vi "Division of Complex Polynomials.vi"(2 "Q":cdb[](array[numeric]) format="%.2f", 3 "P":cdb[](array[numeric]) format="%.2f") -> (0 "Rest":cdb[](array[numeric]) format="%.2f", 1 "P/Q":cdb[](array[numeric]) format="%.2f")   [LabVIEW 2020, in "NI_AdvCtrl_continuous linear.lvlib"]
doc: "LabVIEW no longer supports this VI. You can obtain similar functionality by installing the LabVIEW Simulation Module."
uses:
  <vilib>/addons/control/advanced/NI_AdvCtrl_continuous linear.lvlib
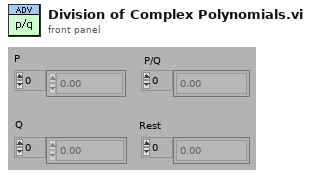
[diagram p1: front panel]
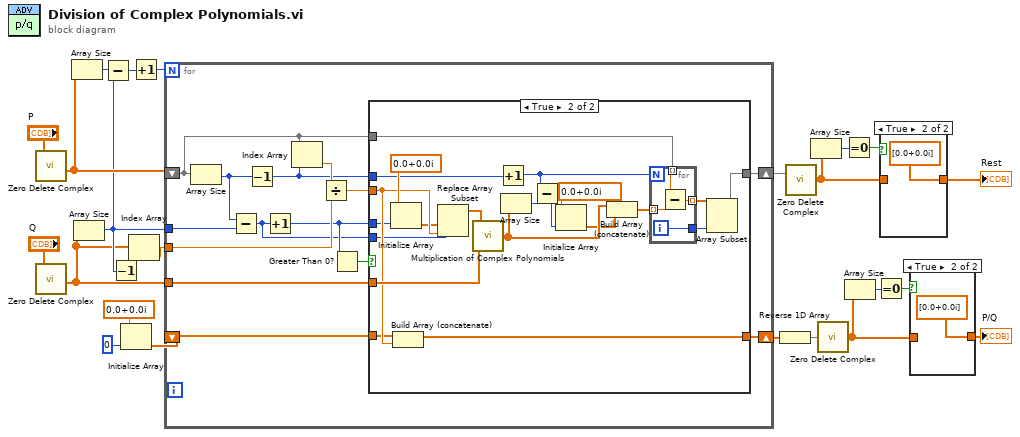
[diagram p0: block diagram]
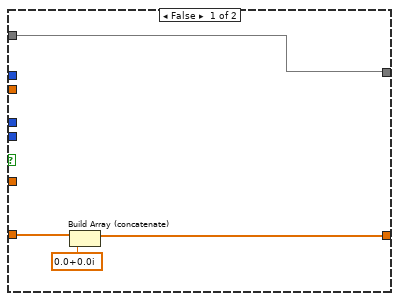
[diagram p4: hidden frame]
diagram:
  n1 = call <vilib>:"Zero Delete Complex.vi"("P"="P") -> ("Q"=w16:cdb[])
  n2 = call <vilib>:"Zero Delete Complex.vi"("P"="Q") -> ("Q"=w10:cdb[])
  n3 = Array Size(array=w16) -> (size(s)=w21:i32)
  n4 = Array Size(array=w10) -> (size(s)=w11:i32)
  n5 = Subtract(x=w21, y=w11) -> (x-y=w14:i32)
  n6 = Decrement(x=w11) -> (x-1=w12:i32)
  n7 = Initialize Array(cdb 0.0+0.0i, 0) -> (w24:cdb[])
  n8 = Index Array(array=w10, index=w12) -> (element=w9:cdb)
  n9 = Increment(x=w14) -> (x+1=w13:i32)
  n10 = for {
    N: w13 -> [_]
    shift-right: [w25] -> w20
    shift-left: w16 -> [w33]
    shift-right: [w26] -> w22
    shift-left: w24 -> [w37]
    tunnel: w10 -> [w34]
    tunnel: w11 -> [w31]
    tunnel: w9 -> [w30]
    n11 = Array Size(array=w33) -> (size(s)=w32:i32)
    n12 = Subtract(x=w32, y=w31) -> (x-y=w27:i32)
    n13 = Decrement(x=w32) -> (x-1=w36:i32)
    n14 = Increment(x=w27) -> (x+1=w29:i32)
    n15 = Index Array(array=w33, index=w36) -> (element=w38:cdb)
    n16 = Divide(x=w38, y=w30) -> (x/y=w35:cdb)
    n17 = Greater Than 0?(x=w29) -> (x > 0?=w28:bool)
    n18 = case shown="True" w28 {
      tunnel: [w42 w51] -> w25
      tunnel: [w39 w63] -> w26
      tunnel: w33 -> [w42 w61]
      tunnel: w29 -> [_ w54]
      tunnel: w34 -> [_ w60]
      tunnel: w35 -> [_ w59]
      tunnel: w36 -> [_ w57]
      tunnel: w37 -> [w41 w56]
      tunnel: w27 -> [_ w53]
      frame False {
        n19 = Build Array (concatenate)(w41, cdb 0.0+0.0i) -> (w39:cdb[])
      }
      frame True {
        n20 = Initialize Array(cdb 0.0+0.0i, w54) -> (w58:cdb[])
        n21 = Build Array (concatenate)(w56, w59) -> (w63:cdb[])
        n22 = Replace Array Subset(array=w58, new element=w59, index=w53) -> (w55:cdb[])
        n23 = call <vilib>:"Multiplication of Complex Polynomials.vi"("Q"=w60, "P"=w55) -> ("P*Q"=w45:cdb[])
        n24 = Increment(x=w57) -> (x+1=w49:i32)
        n25 = Array Size(array=w45) -> (size(s)=w48:i32)
        n26 = Subtract(x=w49, y=w48) -> (x-y=w46:i32)
        n27 = Initialize Array(cdb 0.0+0.0i, w46) -> (w44:cdb[])
        n28 = Build Array (concatenate)(w45, w44) -> (w43:cdb[])
        n29 = for {
          N: w49 -> [_]
          tunnel: w43 -> [w67] mode=indexing
          tunnel: w61 -> [w66] mode=indexing
          tunnel: [w65] -> w50 mode=indexing
          tunnel: [w64] -> w52
          i -> [w64]
          n30 = Subtract(x=w66, y=w67) -> (x-y=w65:cdb)
        }
        n31 = Array Subset(array=w50, length=w52) -> (w51:cdb[])  [unwired: 1 in]
      }
    }
  }
  n32 = Reverse 1D Array(array=w22) -> (reversed array=w19:cdb[])
  n33 = call <vilib>:"Zero Delete Complex.vi"("P"=w20) -> ("Q"=w8:cdb[])
  n34 = Array Size(array=w8) -> (size(s)=w7:i32)
  n35 = call <vilib>:"Zero Delete Complex.vi"("P"=w19) -> ("Q"=w3:cdb[])
  n36 = Equal To 0?(x=w7) -> (x = 0?=w6:bool)
  n37 = Array Size(array=w3) -> (size(s)=w4:i32)
  n38 = Equal To 0?(x=w4) -> (x = 0?=w2:bool)
  n39 = case shown="True" w6 {
    tunnel: w8 -> [w68 _]
    tunnel: [w68 cdb[] [0.0+0.0i] ("rest")] -> w5
    frame False {
    }
    frame True {
    }
  }
  "Rest" <- w5
  n40 = case shown="True" w2 {
    tunnel: [w70 cdb[] [0.0+0.0i] ("rest")] -> w1
    tunnel: w3 -> [w70 _]
    frame False {
    }
    frame True {
    }
  }
  "P/Q" <- w1
